vi "string_parse.vi"(0 "string array":string[](array[string])) -> (2 "f_stop":string, 3 "f_start":string, 4 "f_start double":dbl, 6 "Step di frequenza":string, 8 "Step di frequenza double":dbl, 10 "Ampiezza":string, 12 "f_stop double":dbl, 13 "Ampiezza double":dbl, 14 "Ampiezza string":string)   [LabVIEW 2021]
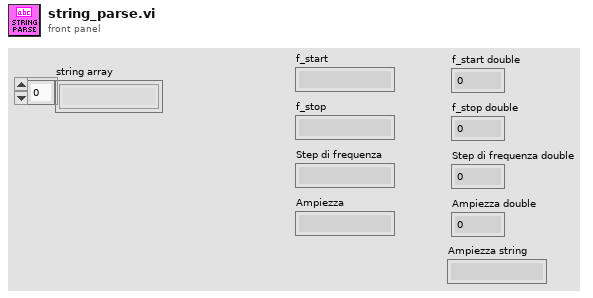
[diagram p1: front panel]
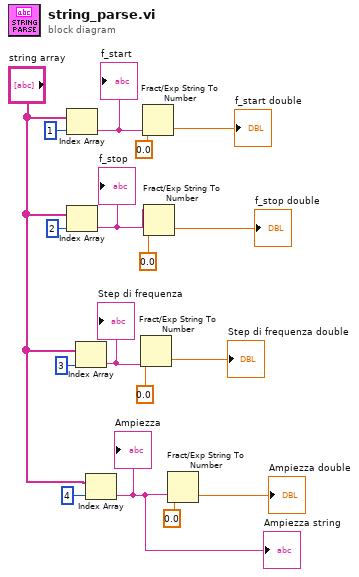
[diagram p0: block diagram]
diagram:
  n1 = Index Array(array="string array", index=1) -> (element=w4:string)
  "f_start" <- w4
  n2 = Index Array(array="string array", index=2) -> (element=w3:string)
  "f_stop" <- w3
  n3 = Index Array(array="string array", index=3) -> (element=w2:string)
  "Step di frequenza" <- w2
  n4 = Index Array(array="string array", index=4) -> (element=w1:string)
  "Ampiezza" <- w1
  "Ampiezza string" <- w1
  n5 = Fract/Exp String To Number(string=w2, default (0 dbl)=0.0) -> (number=→"Step di frequenza double":dbl)  [unwired: 2 in, 1 out]
  n6 = Fract/Exp String To Number(string=w4, default (0 dbl)=0.0) -> (number=→"f_start double":dbl)  [unwired: 2 in, 1 out]
  n7 = Fract/Exp String To Number(string=w3, default (0 dbl)=0.0) -> (number=→"f_stop double":dbl)  [unwired: 2 in, 1 out]
  n8 = Fract/Exp String To Number(string=w1, default (0 dbl)=0.0) -> (number=→"Ampiezza double":dbl)  [unwired: 2 in, 1 out]
